vi "To JSON.vi"(8 "error in":errorcluster, 11 "PDO Mapping in":refnum<class "PDO Mapping.lvclass">) -> (0 "error out":errorcluster, 2 "<JSON>":string, 3 "PDO Mapping out":refnum<class "PDO Mapping.lvclass">)   [LabVIEW 2019, in "PDO Grid.lvlib" / "PDO Mapping.lvclass"]
uses:
  PDO Mapping.lvclass
  Core/OD Entry/OD Entry.lvclass
  PDO Mapping.lvclass/PDO Mapping.ctl
  <vilib>/JDP Science/JSONtext/LVClass Serializer/JSONtext LVClass Serializer.lvclass
  Core/Access Type.ctl
  Core/Electronic Datasheet.lvlib
  6fcefa3a-d29a-4c3f-8950-98bdcb439fc6.vi
  <vilib>/JDP Science/JSONtext/JSONtext.lvlib
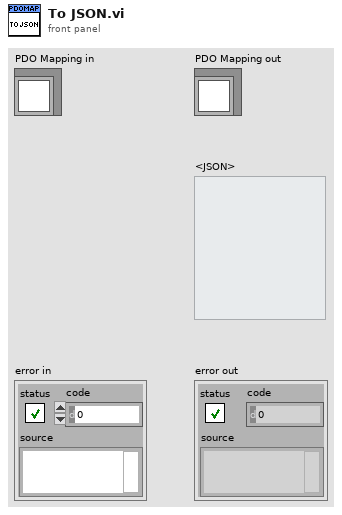
[diagram p1: front panel]
types:
  T1 = typedef "Electronic Datasheet.lvlib/Access Type.ctl" = cluster{"AccessType":enum16{"Ro", "Wo", "Rw", "Const", "Unknown"}, "Null":bool}
  T2 = cluster{"OD Index":u16, "Description":string, "AccessType":T1, "Mapping Targets":refnum<class "OD Entry.lvclass">[], "Dummy Targets":refnum<class "OD Entry.lvclass">[]}
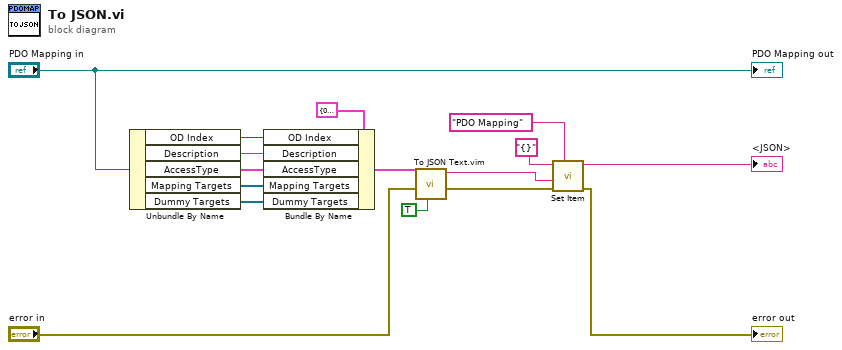
[diagram p0: block diagram]
diagram:
  n1 = Unbundle By Name("PDO Mapping in") -> ("OD Index"=w10:u16, "Description"=w11:string, "AccessType"=w12:T1, "Mapping Targets"=w13:refnum<class "OD Entry.lvclass">[], "Dummy Targets"=w14:refnum<class "OD Entry.lvclass">[])
  n2 = Bundle By Name(cluster=T2 {"OD Index"=0, "Description"="", "AccessType"={"AccessType"=enum."Ro", "Null"=TRUE}, "Mapping Targets"=[], "Dummy Targets"=[]} ("Cluster of class private data"), "OD Index"=w10, "Description"=w11, "AccessType"=w12, "Mapping Targets"=w13, "Dummy Targets"=w14) -> (w9:T2)
  n3 = call "To JSON Text.vim"("Pretty Print?"=TRUE, "error in (no error)"="error in", "Anything"=w9) -> ("error out"=w6:errorcluster, "<JSON>"=w5:string)  [unwired: 7 in]
  n4 = call <vilib>:"Set Item.vi"("$Path or Item Name"="PDO Mapping", "error in (no error)"=w6, "JSON to Insert"=w5, "JSON"="{}") -> ("error out"=→"error out":errorcluster, "<JSON>"=→"<JSON>":string)  [unwired: 4 in, 1 out]
  "PDO Mapping out" <- "PDO Mapping in"
